vi "Send Completion Notification.vi"(7 "Message Priority (Normal)":T2=enum."Normal", 8 "error in (no error)":errorcluster, 9 "Completion Notification Data":T1, 10 "Message Type":refnum<class "Completion Notification Msg.lvclass">, 11 "Message Enqueuer":refnum<class "Message Enqueuer.lvclass">) -> (0 "error out":errorcluster, 3 "Message Enqueuer out":refnum<class "Message Enqueuer.lvclass">)   [LabVIEW 2023, in "Async Methods Actor.lvlib" / "Completion Notification Msg.lvclass"]
doc: "This VI sends the message to an actor."
uses:
  Completion Notification Msg.lvclass
  <vilib>/ActorFramework/Message Enqueuer/Message Enqueuer.lvclass
  <vilib>/ActorFramework/Message Enqueuer/Message Priority.ctl
  C:/Program Files/National Instruments/LabVIEW 2023/vi.lib/ActorFramework/Message/Message.lvclass
  Completion Notification Data.ctl
  Async Message/Async Message.lvclass
  <vilib>/ActorFramework/Message/Message.lvclass
  Completion Notification Msg.lvclass/Completion Notification Msg.ctl
  <vilib>/ActorFramework/Message Enqueuer/Message Enqueuer.lvclass/Message Enqueuer.ctl
  <vilib>/Utility/LVClass/Get LV Class Name.vi
  <resource>/AFDebug/Generate Trace for Message.vi
  <vilib>/ActorFramework/Message Priority Queue/Priority Enqueue.vi
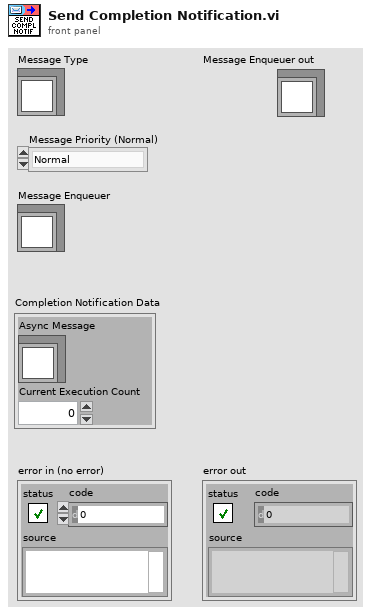
[diagram p1: front panel]
types:
  T1 = typedef "Async Methods Actor.lvlib/Completion Notification Msg.lvclass/Completion Notification Data.ctl" = cluster{"Async Message":refnum<class "Async Message.lvclass">, "Current Execution Count":u32}
  T2 = typedef "Actor Framework.lvlib/Message Enqueuer.lvclass/Message Priority.ctl" = enum16{"Low", "Normal", "High"}
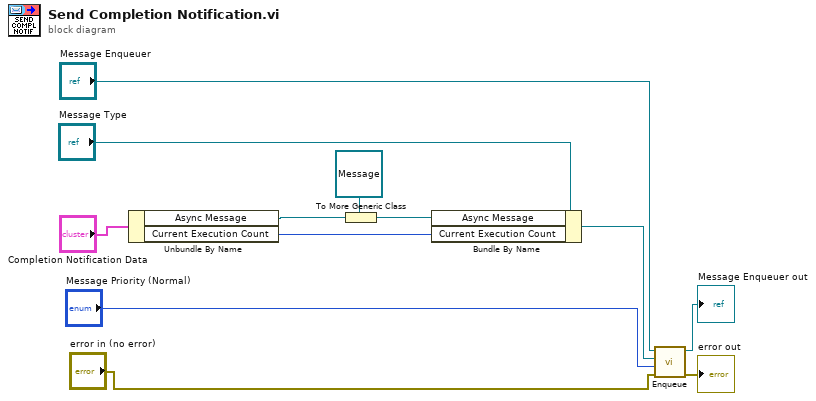
[diagram p0: block diagram]
diagram:
  n1 = Unbundle By Name("Completion Notification Data") -> ("Async Message"=w4:refnum<class "Async Message.lvclass">, "Current Execution Count"=w5:u32)
  n2 = To More Generic Class(target class=refnum<class "Message.lvclass"> refnum ("Async Message"), reference=w4) -> (generic class reference=w2:refnum<class "Message.lvclass">)
  n3 = Bundle By Name(cluster="Message Type", "Async Message"=w2, "Current Execution Count"=w5) -> (w9:refnum<class "Completion Notification Msg.lvclass">)
  n4 = call <vilib>:"Enqueue.vi"("error in (no error)"="error in (no error)", "Message Priority (Normal)"="Message Priority (Normal)", "Message"=w9, "Message Enqueuer in"="Message Enqueuer") -> ("error out"=→"error out":errorcluster, "Message Enqueuer out"=→"Message Enqueuer out":refnum<class "Message Enqueuer.lvclass">)  [unwired: 6 in]
